vi "OAT Get Vector Reference (N Channels).vi"(0 "scaled signals [EU]":waveform(dbl)[](array[waveform]), 1 "reference output mode":T1(ring), 2 "reset? (F)":bool, 5 "speed profile":T2 {"speed [RPM]" format="%.2f"; "time [s]" format="%.2f"}, 7 "pulse/revolution (1)":i32=1, 9 "orders to compensate (1.0)":dbl[](array[numeric])=[1.0] format="%.2f", 11 "error in (no error)":errorcluster, 12 "bandwidth [order]":dbl=1.0 format="%.2f") -> (4 "vector references":cdb[][](array[numeric]) format="%.2f", 15 "error out":errorcluster)   [LabVIEW 2017, in "SoundVib_RefDataProcess.lvlib"]
doc: "Computes the vector references of the specified orders from the slow-roll vibration signals. Use the vector references to compensate shaft bow or runout errors. Wire data to the <B>scaled signal [EU]</B> input to determine the polymorphic instance to use or manually select the instance."
uses:
  <vilib>/addons/Sound and Vibration/Order Analysis/Referece Data Processing/SoundVib_RefDataProcess.lvlib
  <vilib>/addons/Sound and Vibration/Order Analysis/Tach Process/SubVIs/speed profile.ctl
  <vilib>/addons/_NISVFA/_Shared subVIs/Common/svc_Check for Waveform Parameter Continuity (no state).vi
  <vilib>/addons/_NISVFA/_Shared subVIs/Common/svc_Get SV Channel Info.vi
  <vilib>/addons/Sound and Vibration/Order Analysis/Resample Order Tracking/OAT Order Magnitude and Phase (Even Angle Signal, N Channels).vi
  <vilib>/addons/Sound and Vibration/Order Analysis/Resample Order Tracking/OAT Convert to Even Angle Signal (N Channels).vi
  <vilib>/addons/_NISVFA/_Shared subVIs/Common/svc_Engineering Units to Unit Label.vi
  <vilib>/addons/_NISVFA/_Shared subVIs/Common/svc_Unit Label to Engineering Units.vi
  <vilib>/Analysis/NI_AALPro.lvlib
  <vilib>/addons/Sound and Vibration/Order Analysis/Resample Order Tracking/SoundVib_OrderTracking.lvlib
  <vilib>/addons/Sound and Vibration/Order Analysis/Tach Process/SoundVib_TachProcess.lvlib
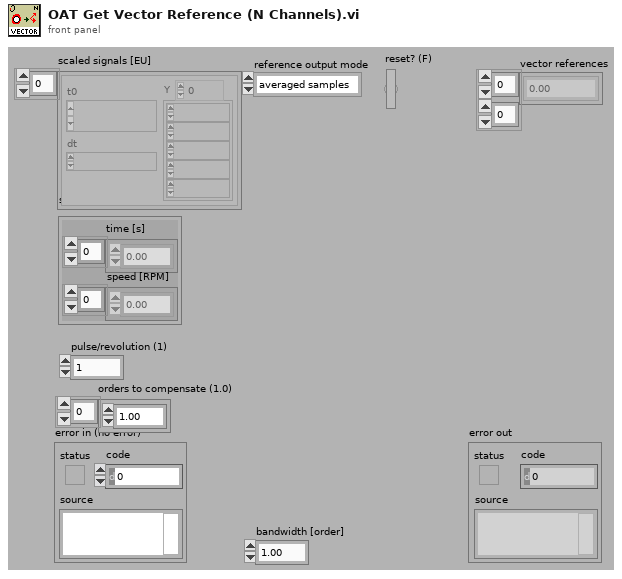
[diagram p1: front panel]
types:
  T1 = enum16{"averaged samples", "initial samples", "final samples"}
  T2 = typedef "SoundVib_TachProcess.lvlib/speed profile.ctl" = cluster{"time [s]":dbl[], "speed [RPM]":dbl[]}
  T3 = cluster{"dt equal":bool, "array length equal":bool, "number channels change":bool}
  T4 = cluster{"dt":bool, "t0 continuity":bool, "array length":bool, "channel info":bool, "name":bool}
  T5 = cluster{"dB on? (T)":bool, "unwrap phase? (T)":bool, "unit in degree? (T)":bool}
  T6 = typedef "svc_Resampled Channel Info.ctl" = cluster{"channel name":string, "description":string, " channel info":T7}
  T7 = typedef "svc_Channel Info.ctl" = cluster{"sensor sensitivity":dbl, "engineering units":T8, "dB reference":dbl, "custom label":string, "weighting filter":T9, "pregain":dbl}
  T8 = typedef "svc_Engineering Units Text Ring.ctl" = u16
  T9 = typedef "svc_Weighting Filter Text Ring.ctl" = u16
  T10 = typedef "OAT Position Info.ctl" = cluster{"positions [s]":dbl[], "samples/rev":dbl}
  T11 = cluster{"time/rev/rpm":dbl[], "magnitude":dbl[]}[][]
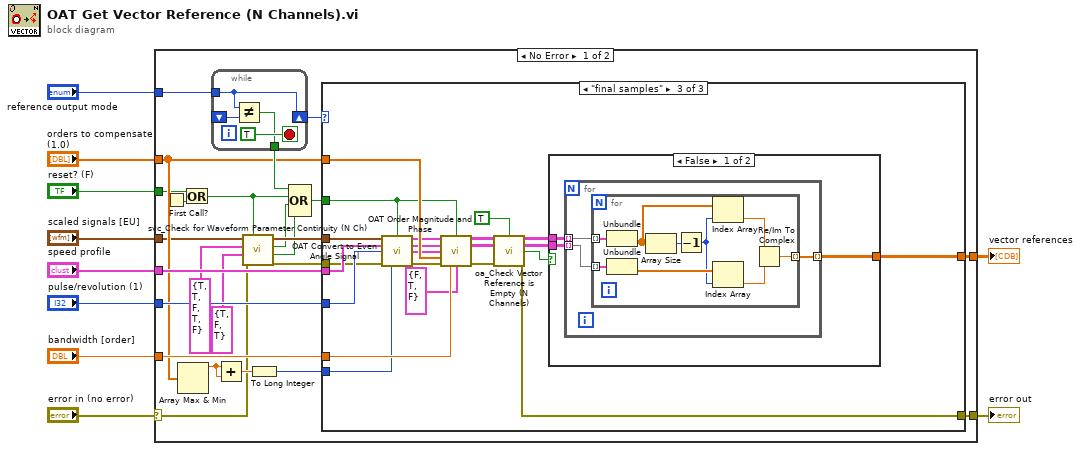
[diagram p0: block diagram]
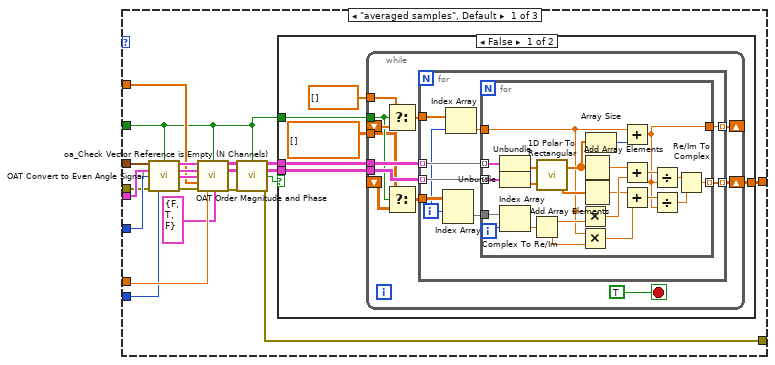
[diagram p2: hidden frame]
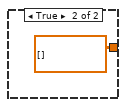
[diagram p3: hidden frame]
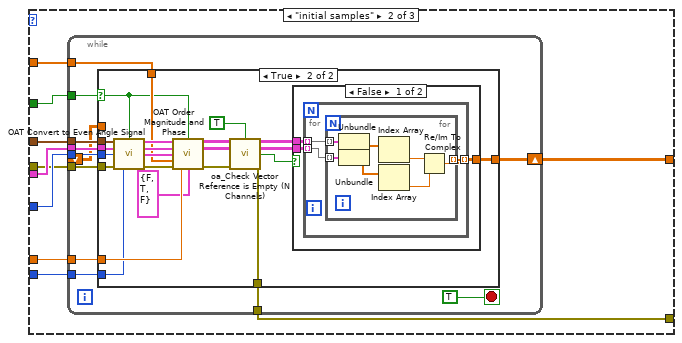
[diagram p4: hidden frame]
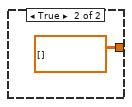
[diagram p6: hidden frame]
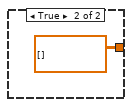
[diagram p7: hidden frame]
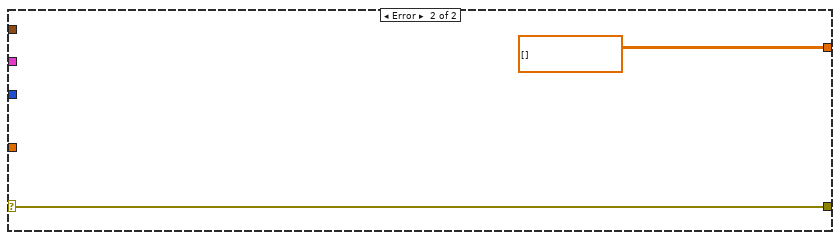
[diagram p8: hidden frame]
diagram:
  n1 = case shown="No Error" "error in (no error)" {
    selector: "error in (no error)" -> [w16 w209]
    tunnel: "scaled signals [EU]" -> [w18 _]
    tunnel: "speed profile" -> [w34 _]
    tunnel: "pulse/revolution (1)" -> [w33 _]
    tunnel: [w32 cdb[][] []] -> w7
    tunnel: [w31 w209] -> w6
    tunnel: "bandwidth [order]" -> [w30 _]
    tunnel: "orders to compensate (1.0)" -> [w23 _]
    tunnel: "reference output mode" -> [w29 _]
    tunnel: "reset? (F)" -> [w20 _]
    frame No Error {
      n2 = First Call?() -> (First Call?: T/F=w21:bool)
      n3 = Array Max & Min(array=w23) -> (max value=w25:dbl)  [unwired: 3 out]
      n4 = Or(x=w20, y=w21) -> (x .or. y?=w19:bool)
      n5 = while {
        shift-right: [w38] -> w28
        shift-left: _ -> [w37]
        tunnel: w29 -> [w38]
        tunnel: [w35] -> w27
        stop <- TRUE stop-if-true
        n6 = Not Equal?(x=w38, y=w37) -> (x != y?=w35:bool)
      }
      n7 = Add(x=w25, y=w25) -> (x+y=w24:dbl)
      n8 = call <vilib>:"svc_Check for Waveform Parameter Continuity (N Ch).vi"("restart averaging (F)"=w19, "error in (no error)"=w16, "checks for multichannel parameters"=T3 {"dt equal"=TRUE, "array length equal"=FALSE, "number channels change"=TRUE}, "checks for channel parameter change"=T4 {"dt"=TRUE, "t0 continuity"=TRUE, "array length"=FALSE, "channel info"=TRUE, "name"=FALSE}, "scaled signal(s)"=w18) -> ("error out"=w15:errorcluster, "multichannel parameter changed"=w13:bool, "waveform parameter changed"=w14:bool, "dup scaled signal(s)"=w17:waveform(dbl)[])  [unwired: 3 out]
      n9 = To Long Integer(number=w24) -> (32bit integer=w22:i32)
      n10 = Compound Arithmetic op=OR(w27, w19, w14, w13) -> (w26:bool)
      n11 = case shown="\"final samples\"" w28 {
        tunnel: w17 -> [w59 w120 w192]
        tunnel: w34 -> [w58 w119 w191]
        tunnel: w33 -> [w57 w118 w190]
        tunnel: w15 -> [w56 w117 w189]
        tunnel: [w49 w116 w188] -> w32
        tunnel: [w41 w111 w173] -> w31
        tunnel: w30 -> [w51 w115 w187]
        tunnel: w23 -> [w50 w114 w186]
        tunnel: w26 -> [w39 w113 w179]
        tunnel: w22 -> [w48 w112 w181]
        frame "averaged samples", Default {
          n12 = call-poly <vilib>:"OAT Convert to Even Angle Signal.vi"("scaled signals [EU]"=w59, "reset? (F)"=w39, "speed profile"=w58, "pulse/revolution (1)"=w57, "error in (no error)"=w56, "max order (auto)"=w48) -> ("even-angle signals"=w55:cluster{"r0":dbl, "dr":dbl, "Y":dbl[]}[], "even-angle channel info"=w54:T6[], "even-angle position info"=w53:T10, "error out"=w52:errorcluster)  [unwired: 5 in, 1 out]
          n13 = call-poly <vilib>:"OAT Order Magnitude and Phase.vi"("even-angle signals"=w55, "reset? (F)"=w39, "even-angle channel info"=w54, "even-angle position info"=w53, "orders to compute (1.0)"=w50, "error in (no error)"=w52, "bandwidth [order]"=w51, "view"=T5 {"dB on? (T)"=FALSE, "unwrap phase? (T)"=TRUE, "unit in degree? (T)"=FALSE}) -> ("magnitudes [RMS]"=w46:T11, "phases [phase lag]"=w45:cluster{"time/rev/rpm":dbl[], "phase":dbl[]}[][], "error out"=w42:errorcluster)  [unwired: 2 in, 3 out]
          n14 = call <vilib>:"oa_Check Vector Reference is Empty (N Channels).vi"("magnitudes [RMS] in"=w46, "reset? (F)"=w39, "phases [phase lag] in"=w45, "error in (no error)"=w42) -> ("magnitudes [RMS] out"=w44:T11, "phases [phase lag] out"=w43:cluster{"time/rev/rpm":dbl[], "phase":dbl[]}[][], "empty?"=w40:bool, "error out"=w41:errorcluster)  [unwired: 8 in]
          n15 = case shown="False" w40 {
            tunnel: [w65 cdb[][] []] -> w49
            tunnel: w39 -> [w62 _]
            tunnel: w44 -> [w61 _]
            tunnel: w43 -> [w60 _]
            frame False {
              n16 = while {
                tunnel: w61 -> [w77]
                tunnel: w60 -> [w76]
                shift-right: [w73] -> _
                shift-left: _ -> [w72]
                shift-right: [w74] -> w65
                shift-left: _ -> [w70]
                tunnel: w62 -> [w68]
                tunnel: dbl[] [] -> [w69]
                tunnel: cdb[][] [] -> [w66]
                stop <- TRUE stop-if-true
                n17 = Select(t=w69, s=w68, f=w72) -> (s? t:f=w71:dbl[])
                n18 = Select(t=w66, s=w68, f=w70) -> (s? t:f=w67:cdb[][])
                n19 = for {
                  tunnel: w77 -> [w86] mode=indexing
                  tunnel: w76 -> [w85] mode=indexing
                  tunnel: [w84] -> w74 mode=indexing
                  tunnel: [w83] -> w73 mode=indexing
                  tunnel: w71 -> [w80]
                  tunnel: w67 -> [w82]
                  i -> [w79]
                  n20 = Index Array(array=w82, index (row)=w79) -> (element=w81:cdb[])  [unwired: 1 in]
                  n21 = Index Array(array=w80, index=w79) -> (element=w78:dbl)
                  n22 = for {
                    tunnel: w86 -> [w109] mode=indexing
                    tunnel: w85 -> [w108] mode=indexing
                    tunnel: [w106] -> w84 mode=indexing
                    tunnel: [w93] -> w83
                    tunnel: w81 -> [w90]
                    tunnel: w78 -> [w87]
                    i -> [w88]
                    n23 = Unbundle(w109) -> ("magnitude"=w107:dbl[])  [unwired: 1 out]
                    n24 = Unbundle(w108) -> ("phase"=w105:dbl[])  [unwired: 1 out]
                    n25 = Index Array(array=w90, index=w88) -> (element=w89:cdb)
                    n26 = Complex To Re/Im(x + iy=w89) -> (x=w103:dbl, y=w102:dbl)
                    n27 = call <vilib>:"1D Polar To Rectangular.vi"("Magnitude"=w107, "Phase"=w105) -> ("X"=w101:dbl[], "Y"=w100:dbl[])  [unwired: 1 out]
                    n28 = Multiply(x=w87, y=w103) -> (x*y=w98:dbl)
                    n29 = Multiply(x=w87, y=w102) -> (x*y=w96:dbl)
                    n30 = Add Array Elements(numeric array=w101) -> (sum=w99:dbl)
                    n31 = Add Array Elements(numeric array=w100) -> (sum=w97:dbl)
                    n32 = Array Size(array=w101) -> (size(s)=w104:i32)
                    n33 = Add(x=w87, y=w104) -> (x+y=w93:dbl)
                    n34 = Add(x=w99, y=w98) -> (x+y=w95:dbl)
                    n35 = Add(x=w97, y=w96) -> (x+y=w94:dbl)
                    n36 = Divide(x=w95, y=w93) -> (x/y=w92:dbl)
                    n37 = Divide(x=w94, y=w93) -> (x/y=w91:dbl)
                    n38 = Re/Im To Complex(1:w91, 2:w92) -> (0:w106:cdb)
                  }
                }
              }
            }
            frame True {
            }
          }
        }
        frame "initial samples" {
          n39 = while {
            tunnel: w120 -> [w132]
            tunnel: w119 -> [w131]
            tunnel: w118 -> [w130]
            tunnel: w117 -> [w129]
            tunnel: w115 -> [w127]
            tunnel: w114 -> [w126]
            tunnel: w113 -> [w125]
            shift-right: [w128] -> w116
            shift-left: _ -> [w123]
            tunnel: w112 -> [w122]
            tunnel: [w121] -> w111
            stop <- TRUE stop-if-true
            n40 = case shown="True" w125 {
              selector: w125 -> [_ w143]
              tunnel: w132 -> [_ w156]
              tunnel: w131 -> [_ w155]
              tunnel: w130 -> [_ w154]
              tunnel: w129 -> [w133 w153]
              tunnel: [w134 w148] -> w128
              tunnel: w127 -> [_ w147]
              tunnel: w126 -> [_ w146]
              tunnel: w123 -> [w134 _]
              tunnel: w122 -> [_ w145]
              tunnel: [w133 w137] -> w121
              frame False {
              }
              frame True {
                n41 = call-poly <vilib>:"OAT Convert to Even Angle Signal.vi"("scaled signals [EU]"=w156, "reset? (F)"=w143, "speed profile"=w155, "pulse/revolution (1)"=w154, "error in (no error)"=w153, "max order (auto)"=w145) -> ("even-angle signals"=w152:cluster{"r0":dbl, "dr":dbl, "Y":dbl[]}[], "even-angle channel info"=w151:T6[], "even-angle position info"=w150:T10, "error out"=w149:errorcluster)  [unwired: 5 in, 1 out]
                n42 = call-poly <vilib>:"OAT Order Magnitude and Phase.vi"("even-angle signals"=w152, "reset? (F)"=w143, "even-angle channel info"=w151, "even-angle position info"=w150, "orders to compute (1.0)"=w146, "error in (no error)"=w149, "bandwidth [order]"=w147, "view"=T5 {"dB on? (T)"=FALSE, "unwrap phase? (T)"=TRUE, "unit in degree? (T)"=FALSE}) -> ("magnitudes [RMS]"=w141:T11, "phases [phase lag]"=w140:cluster{"time/rev/rpm":dbl[], "phase":dbl[]}[][], "error out"=w142:errorcluster)  [unwired: 2 in, 3 out]
                n43 = call <vilib>:"oa_Check Vector Reference is Empty (N Channels).vi"("magnitudes [RMS] in"=w141, "reset? (F)"=TRUE, "phases [phase lag] in"=w140, "error in (no error)"=w142) -> ("magnitudes [RMS] out"=w139:T11, "phases [phase lag] out"=w138:cluster{"time/rev/rpm":dbl[], "phase":dbl[]}[][], "empty?"=w136:bool, "error out"=w137:errorcluster)  [unwired: 8 in]
                n44 = case shown="False" w136 {
                  tunnel: [w159 cdb[][] []] -> w148
                  tunnel: w139 -> [w158 _]
                  tunnel: w138 -> [w157 _]
                  frame False {
                    n45 = for {
                      tunnel: w158 -> [w162] mode=indexing
                      tunnel: w157 -> [w161] mode=indexing
                      tunnel: [w160] -> w159 mode=indexing
                      n46 = for {
                        tunnel: w162 -> [w169] mode=indexing
                        tunnel: w161 -> [w168] mode=indexing
                        tunnel: [w167] -> w160 mode=indexing
                        n47 = Unbundle(w169) -> ("magnitude"=w166:dbl[])  [unwired: 1 out]
                        n48 = Unbundle(w168) -> ("phase"=w165:dbl[])  [unwired: 1 out]
                        n49 = Index Array(array=w166) -> (element=w164:dbl)  [unwired: 1 in]
                        n50 = Index Array(array=w165) -> (element=w163:dbl)  [unwired: 1 in]
                        n51 = Re/Im To Complex(1:w163, 2:w164) -> (0:w167:cdb)
                      }
                    }
                  }
                  frame True {
                  }
                }
              }
            }
          }
        }
        frame "final samples" {
          n52 = call-poly <vilib>:"OAT Convert to Even Angle Signal.vi"("scaled signals [EU]"=w192, "reset? (F)"=w179, "speed profile"=w191, "pulse/revolution (1)"=w190, "error in (no error)"=w189, "max order (auto)"=w181) -> ("even-angle signals"=w185:cluster{"r0":dbl, "dr":dbl, "Y":dbl[]}[], "even-angle channel info"=w184:T6[], "even-angle position info"=w183:T10, "error out"=w182:errorcluster)  [unwired: 5 in, 1 out]
          n53 = call-poly <vilib>:"OAT Order Magnitude and Phase.vi"("even-angle signals"=w185, "reset? (F)"=w179, "even-angle channel info"=w184, "even-angle position info"=w183, "orders to compute (1.0)"=w186, "error in (no error)"=w182, "bandwidth [order]"=w187, "view"=T5 {"dB on? (T)"=FALSE, "unwrap phase? (T)"=TRUE, "unit in degree? (T)"=FALSE}) -> ("magnitudes [RMS]"=w178:T11, "phases [phase lag]"=w176:cluster{"time/rev/rpm":dbl[], "phase":dbl[]}[][], "error out"=w174:errorcluster)  [unwired: 2 in, 3 out]
          n54 = call <vilib>:"oa_Check Vector Reference is Empty (N Channels).vi"("magnitudes [RMS] in"=w178, "reset? (F)"=TRUE, "phases [phase lag] in"=w176, "error in (no error)"=w174) -> ("magnitudes [RMS] out"=w177:T11, "phases [phase lag] out"=w175:cluster{"time/rev/rpm":dbl[], "phase":dbl[]}[][], "empty?"=w172:bool, "error out"=w173:errorcluster)  [unwired: 8 in]
          n55 = case shown="False" w172 {
            tunnel: [w195 cdb[][] []] -> w188
            tunnel: w177 -> [w194 _]
            tunnel: w175 -> [w193 _]
            frame False {
              n56 = for {
                tunnel: w194 -> [w198] mode=indexing
                tunnel: w193 -> [w197] mode=indexing
                tunnel: [w196] -> w195 mode=indexing
                n57 = for {
                  tunnel: w198 -> [w207] mode=indexing
                  tunnel: w197 -> [w206] mode=indexing
                  tunnel: [w205] -> w196 mode=indexing
                  n58 = Unbundle(w207) -> ("magnitude"=w200:dbl[])  [unwired: 1 out]
                  n59 = Unbundle(w206) -> ("phase"=w204:dbl[])  [unwired: 1 out]
                  n60 = Array Size(array=w200) -> (size(s)=w201:i32)
                  n61 = Decrement(x=w201) -> (x-1=w199:i32)
                  n62 = Index Array(array=w200, index=w199) -> (element=w203:dbl)
                  n63 = Index Array(array=w204, index=w199) -> (element=w202:dbl)
                  n64 = Re/Im To Complex(1:w202, 2:w203) -> (0:w205:cdb)
                }
              }
            }
            frame True {
            }
          }
        }
      }
    }
    frame Error {
    }
  }
  "error out" <- w6
  "vector references" <- w7
